vi "SIM_Pressure.vi"(8 "Zero Pressure\n(F = leave as is)":bool, 9 "Pressure Offset":dbl format="%.2f", 10 "sim_low":dbl format="%.2f", 11 "sim_high":dbl=1.0 format="%.2f") -> (3 "Pressure":dbl format="%.2f")   [LabVIEW 2016]
panel:
  in  "constant value":dbl=1.0 format="%.2f"
  in  "Return constant value":bool
  # "ON"
  # "OFF"
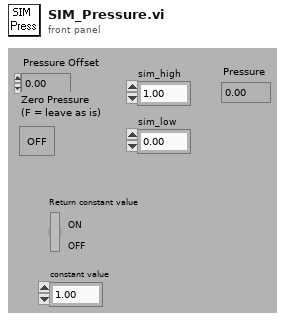
[diagram p1: front panel]
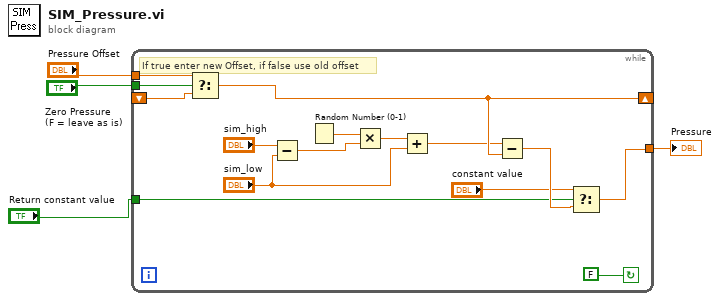
[diagram p0: block diagram]
diagram:
  n1 = while {
    tunnel: "Return constant value" -> [w6]
    tunnel: "Zero Pressure\n(F = leave as is)" -> [w17]
    tunnel: "Pressure Offset" -> [w18]
    shift-left: _ -> [w19]
    shift-right: [w15] -> _
    tunnel: [w5] -> w4
    stop <- FALSE continue-if-true
    # "If true enter new Offset, if false use old offset"
    n2 = Select(t=w18, s=w17, f=w19) -> (s? t:f=w15:dbl)
    n3 = Subtract(x="sim_high", y="sim_low") -> (x-y=w12:dbl)
    n4 = Random Number (0-1)() -> (number: 0 to 1=w13:dbl)
    n5 = Multiply(x=w13, y=w12) -> (x*y=w11:dbl)
    n6 = Add(x=w11, y="sim_low") -> (x+y=w9:dbl)
    n7 = Subtract(x=w9, y=w15) -> (x-y=w8:dbl)
    n8 = Select(t="constant value", s=w6, f=w8) -> (s? t:f=w5:dbl)
  }
  "Pressure" <- w4
